vi "grabWindow.vi"(4 "w (-1)":i32=-1, 6 "y (0)":i32, 7 "h (-1)":i32=-1, 8 "Error In":errorcluster, 9 "x (0)":i32, 10 "window (0)":u64, 11 "QScreen In":refnum<class "QScreen.lvclass">) -> (0 "Error Out":errorcluster, 2 "Value":refnum<class "QPixmap.lvclass">, 3 "QScreen Out":refnum<class "QScreen.lvclass">)   [LabVIEW 2014, in "QScreen.lvclass"]
doc: "LabVIEW-specific documentation is not yet available. See <b>https://doc.qt.io/qt-5/qscreen.html#grabWindow</b>"
uses:
  QScreen.lvclass
  QPixmap/QPixmap.lvclass
  LQ Core/LQIdentity/LQIdentity.lvclass/LQIdentity.ctl
  LQ Core/LQSerialData/LQSerialData.lvclass/LQSerialData.ctl
  LQ Core/LQ Core.lvlib
  LQ Core/LQIdentity/LQIdentity.lvclass
  LQ Core/LQSerialData/LQSerialData.lvclass
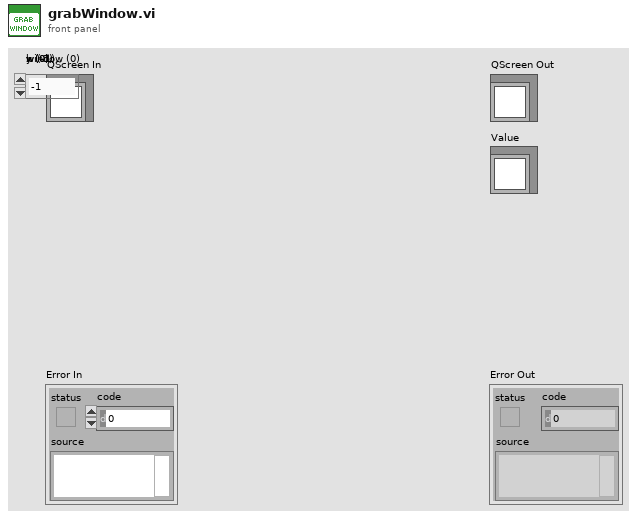
[diagram p1: front panel]
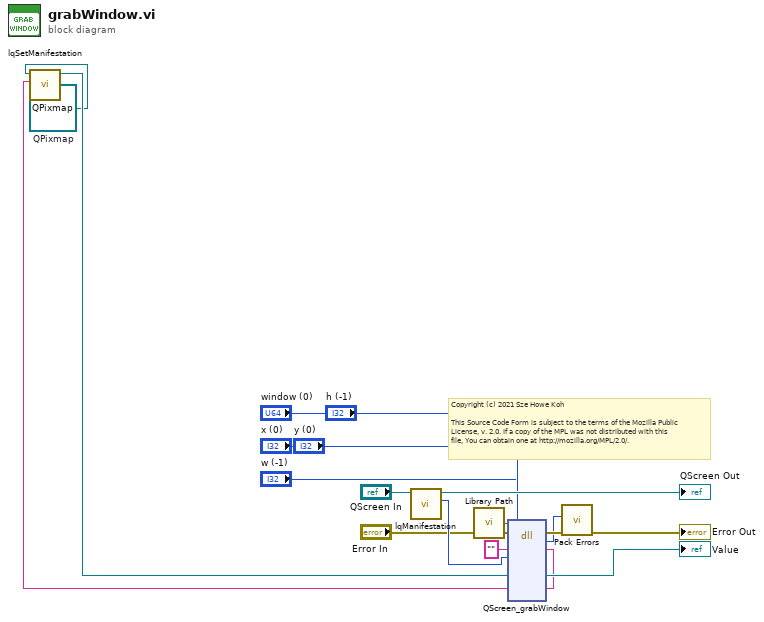
[diagram p0: block diagram]
diagram:
  w6 = refnum<class "QPixmap.lvclass"> refnum  # QPixmap
  # "Copyright (c) 2021 Sze Howe Koh\n\nThis Source Code Form is subject to the terms of the Mozilla Public\nLicense, v. 2.0. If a copy of the MPL was not distributed with this\nfile, You can obtain one at http://mozilla.org/MPL/2.0/."
  n1 = call "lqManifestation.vi"("LQIdentity in"="QScreen In") -> ("Manifestation"=w13:u64, "LQIdentity out"=→"QScreen Out":refnum<class "QScreen.lvclass">)  [unwired: 9 in]
  n2 = call "Library Path.vi"() -> ("Library Path"=w14:path)
  n3 = dll-call lib="?" fn="QScreen_grabWindow"(path in=w14, error in="Error In", "_retVal"="" ("retVal"), "_instance"=w13, "window"="window (0)", "x"="x (0)", "y"="y (0)", "w"="w (-1)", "h"="h (-1)") -> (error out=w11:errorcluster, w9:i32, "_retVal"=w7:string)  [unwired: 7 in, 1 out]
  n4 = call "lqSetManifestation.vi"("Manifestation"=w7, "LQSerialData in"=w6) -> ("LQSerialData out"=→"Value":refnum<class "QPixmap.lvclass">)  [unwired: 8 in, 1 out]
  n5 = call "Pack Errors.vi"("Error In"=w11, "Error Code"=w9) -> ("Error Out"=→"Error Out":errorcluster)  [unwired: 9 in]
